vi "串口数据采集.vi"() -> ()   [LabVIEW 2014]
uses:
  <vilib>/Instr/_visa.llb/VISA Configure Serial Port (Instr).vi
panel:
  out "帮助文档":string="               系统使用说明\n     欢迎使用LabVIEW温度监控系统V3.0！\n      ①程序运行时此帮助文档5秒后会自动关闭。\n      ②程序运行前请先正确配置串口号。\n      ③采样周期默认为1000ms，可根据需要在线设置，但建议不低于500。\n      ④状态及数据区显示系统运行的各种状态或采集的原始数据；时间记录区显示的分别是系统已运行的时间及系统开始运行的起始时刻。\n      ⑤默认的温度上下限分别为25℃和15℃，可随时根据实际情况修改，温度超过设定界限对应指示灯会闪烁并伴有蜂鸣器警告。\n      ⑥设置的快捷键：串口开关按钮<Shift+F1>,帮助按钮<Home>，停止按钮<End>，退出按钮<Delete>。\n      \n"
  in  "帮助":bool
  in  "退出":bool
  in  "停止":bool
  out "状态及数据":string="程序待运行……"
  out "数据采集量":dbl format="%06.0f"
  out "0CH":dbl format="%.2g"
  out "1CH":dbl format="%.2f"
  out "2CH":dbl format="%.2g"
  out "运行时间":string="0  00:00:00"
  out "开始时刻":string="2017/1/1 00:00:00"
  out "低温":bool
  out "高温":bool
  out "2CH":bool
  out "1CH":bool
  out "0CH":bool
  in  "串口开关":bool
  in  "低温限":dbl=15.0 format="%.1g"
  in  "高温限":dbl=25.0 format="%.1f"
  in  "起始号":dbl format="%0#6.0p"
  in  "周期":u32=1000
  in  "端口":refnum<visa-resource-name>="COM2" caption="端口号"
  out "温度曲线":dynamicdata(graph)
  # "LabVIEW温度监控系统V3.0"
  # "串口配置"
  # "采样周期"
  # "时间记录"
  # "数据采集量"
  # "超限报警"
  # "状态及数据"
  # "数值显示"
  # "退出"
  # "停止"
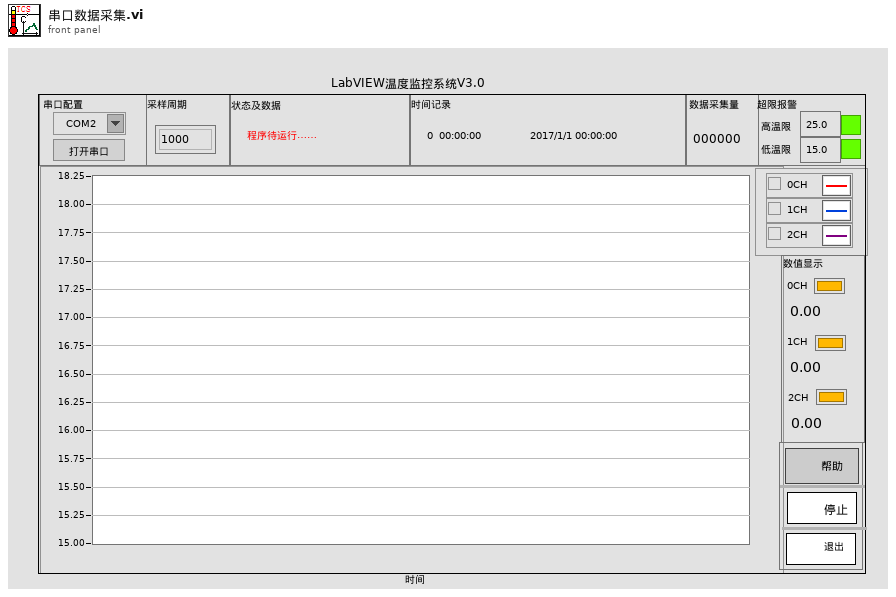
[diagram p1: front panel]
types:
  T1 = enum8{"Enabled", "Disabled", "Disabled and Grayed Out"}
  T2 = enum16{"open", "replace", "create", "open or create", "replace or create", "replace or create with confirmation"}
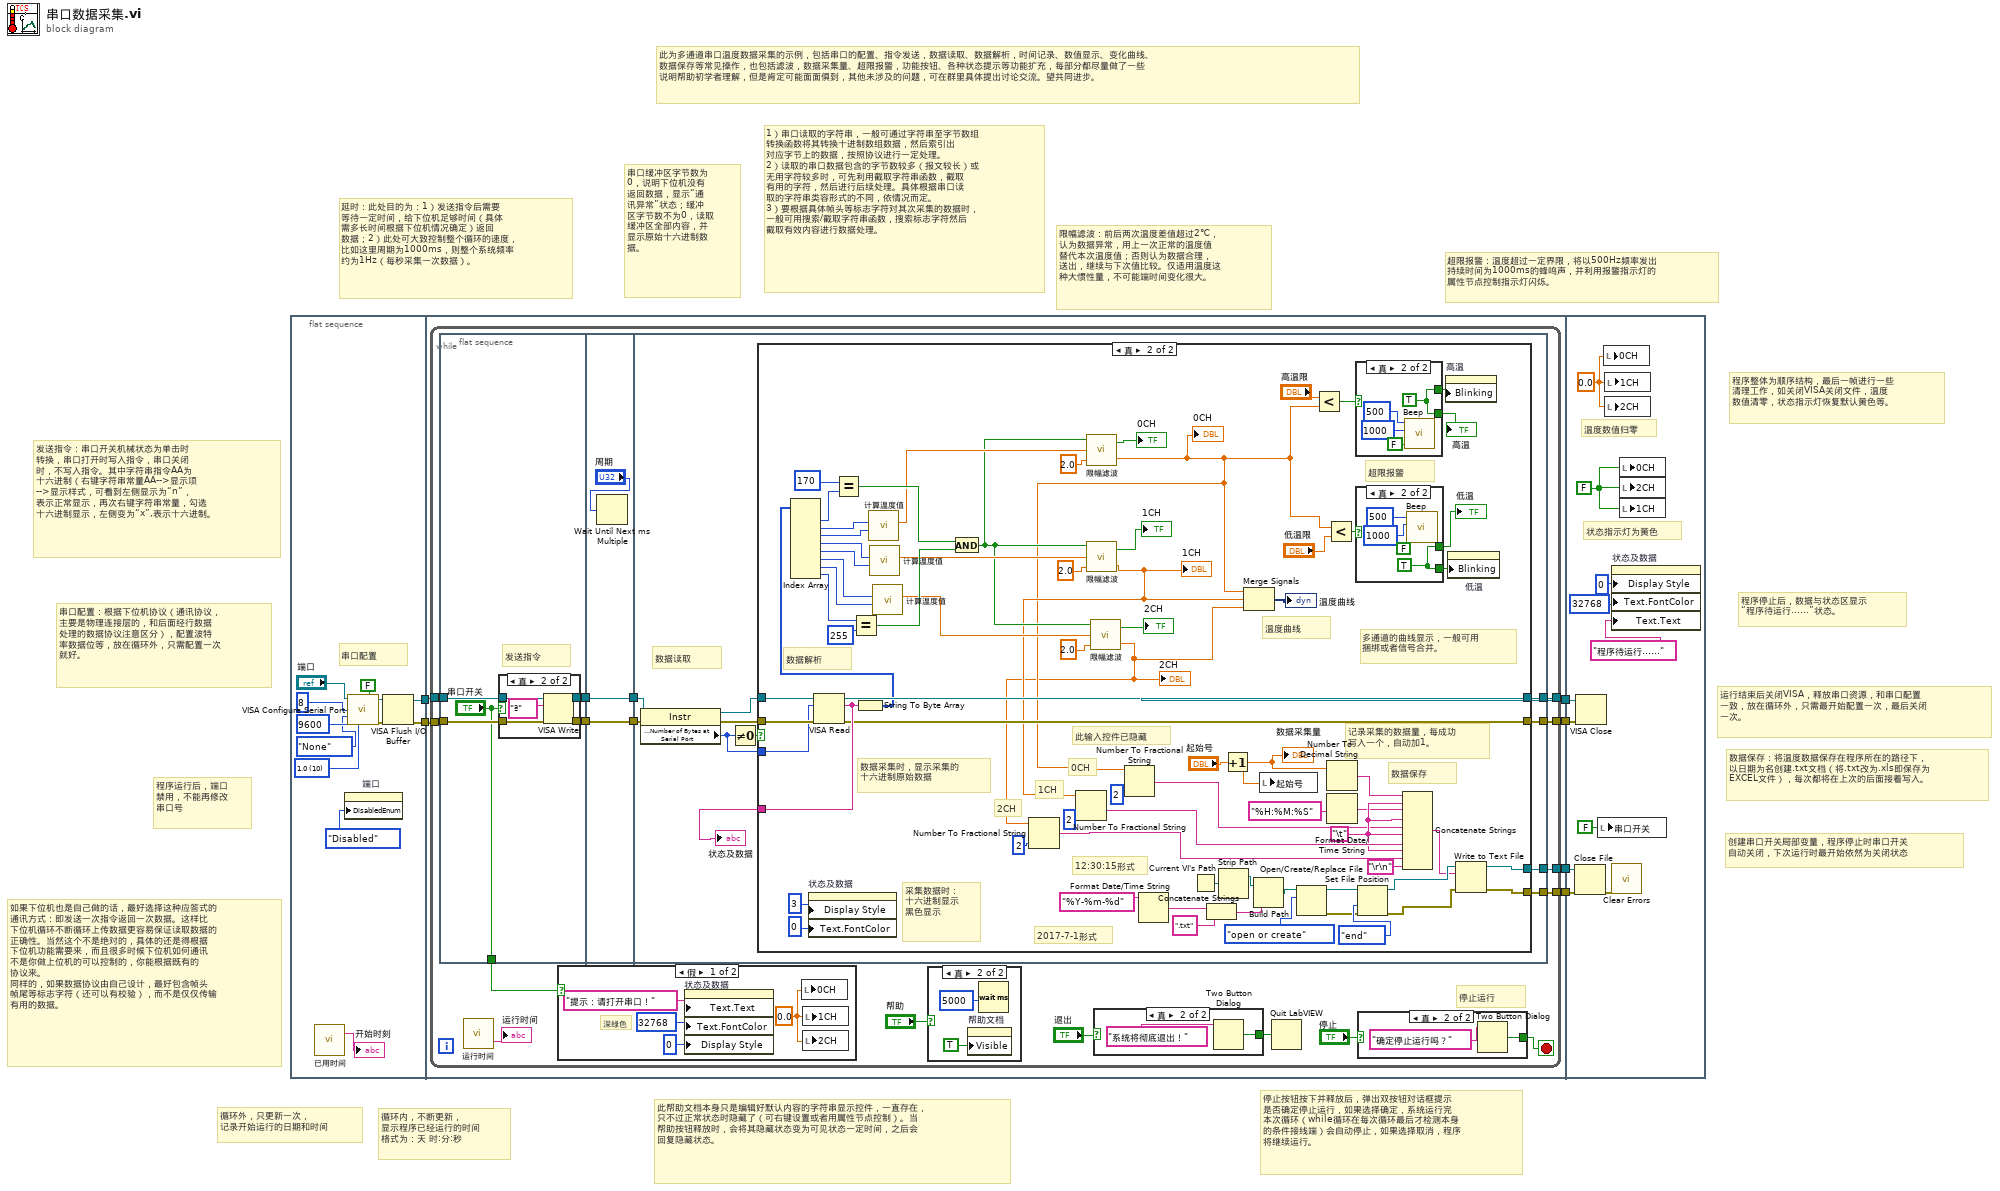
[diagram p0: block diagram]
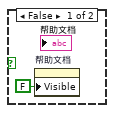
[diagram p2: hidden frame]
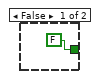
[diagram p3: hidden frame]
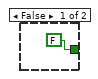
[diagram p5: hidden frame]
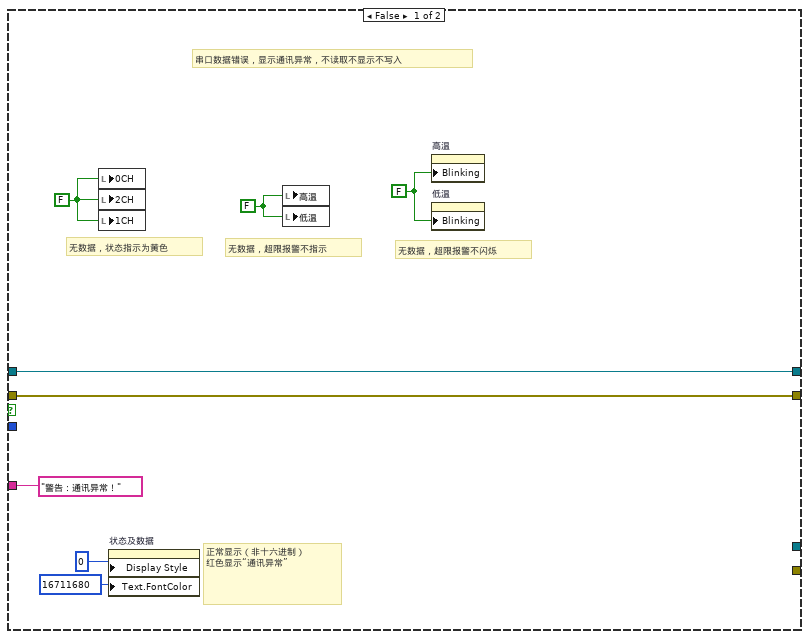
[diagram p7: hidden frame]
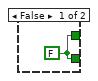
[diagram p8: hidden frame]
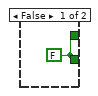
[diagram p9: hidden frame]
diagram:
  # "此为多通道串口温度数据采集的示例，包括串口的配置、指令发送，数据读取、数据解析，时间记录、数值显示、变化曲线、\n数据保存等常见操作，也包括滤波，数据采集量、超限报警，功能按钮、各种状态提示等功能扩充，每部分都尽量做了一些\n说明帮助初学者理解，但是肯定可能面面俱到，其他未涉及的问题，可在群里具体提出讨论交流。望共同进步。"
  # "程序整体为顺序结构，最后一帧进行一些\n清理工作，如关闭VISA关闭文件，温度\n数值清零，状态指示灯恢复默认黄色等。"
  # "创建串口开关局部变量，程序停止时串口开关\n自动关闭，下次运行时最开始依然为关闭状态"
  # "如果下位机也是自己做的话，最好选择这种应答式的\n通讯方式：即发送一次指令返回一次数据。这样比\n下位机循环不断循环上传数据更容易保证读取数据的\n正确性。当然这个不是绝对的，具体的还是得根据\n下位机功能需要来，而且很多时候下位机如何通讯\n不是你做上位机的可以控制的，你能根据既有的\n协议来。\n同样的，如果数据协议由自己设计，最好包含帧头\n帧尾等标志字符（还可以有校验），而不是仅仅传输\n有用的数据。"
  # "1）串口读取的字符串，一般可通过字符串至字节数组\n转换函数将其转换十进制数组数据，然后索引出\n对应字节上的数据，按照协议进行一定处理。\n2）读取的串口数据包含的字节数较多（报文较长）或\n无用字符较多时，可先利用截取字符串函数，截取\n有用的字符，然后进行后续处理。具体根据串口读\n取的字符串类容形式的不同，依情况而定。\n3）要根据具体帧头等标志字符对其次采集的数据时，\n一般可用搜索/截取字符串函数，搜索标志字符然后\n截取有效内容进行数据处理。"
  # "程序停止后，数据与状态区显示\n“程序待运行……”状态。"
  # "串口缓冲区字节数为\n0，说明下位机没有\n返回数据，显示“通\n讯异常”状态；缓冲\n区字节数不为0，读取\n缓冲区全部内容，并\n显示原始十六进制数\n据。"
  # "运行结束后关闭VISA，释放串口资源，和串口配置\n一致，放在循环外，只需最开始配置一次，最后关闭\n一次。"
  # "数据保存：将温度数据保存在程序所在的路径下，\n以日期为名创建.txt文档（将.txt改为.xls即保存为\nEXCEL文件），每次都将在上次的后面接着写入。"
  # "超限报警：温度超过一定界限，将以500Hz频率发出\n持续时间为1000ms的蜂鸣声，并利用报警指示灯的\n属性节点控制指示灯闪烁。"
  # "停止按钮按下并释放后，弹出双按钮对话框提示\n是否确定停止运行，如果选择确定，系统运行完\n本次循环（while循环在每次循环最后才检测本身\n的条件接线端）会自动停止，如果选择取消，程序\n将继续运行。"
  # "此帮助文档本身只是编辑好默认内容的字符串显示控件，一直存在，\n只不过正常状态时隐藏了（可右键设置或者用属性节点控制）。当\n帮助按钮释放时，会将其隐藏状态变为可见状态一定时间，之后会\n回复隐藏状态。"
  # "延时：此处目的为：1）发送指令后需要\n等待一定时间，给下位机足够时间（具体\n需多长时间根据下位机情况确定）返回\n数据；2）此处可大致控制整个循环的速度，\n比如这里周期为1000ms，则整个系统频率\n约为1Hz（每秒采集一次数据）。"
  # "发送指令：串口开关机械状态为单击时\n转换，串口打开时写入指令，串口关闭\n时，不写入指令。其中字符串指令AA为\n十六进制（右键字符串常量AA-->显示项\n-->显示样式，可看到左侧显示为“n”，\n表示正常显示，再次右键字符串常量，勾选\n十六进制显示，左侧变为“x”,表示十六进制。"
  # "串口配置：根据下位机协议（通讯协议，\n主要是物理连接层的，和后面经行数据\n处理的数据协议注意区分），配置波特\n率数据位等，放在循环外，只需配置一次\n就好。"
  # "程序运行后，端口\n禁用，不能再修改\n串口号"
  # "限幅滤波：前后两次温度差值超过2℃，\n认为数据异常，用上一次正常的温度值\n替代本次温度值；否则认为数据合理，\n送出，继续与下次值比较。仅适用温度这\n种大惯性量，不可能端时间变化很大。"
  # "循环内，不断更新，\n显示程序已经运行的时间\n格式为：天 时:分:秒"
  # "循环外，只更新一次，\n记录开始运行的日期和时间"
  n1 = flat-sequence {
    tunnel: [w12] -> w6
    tunnel: [w13] -> w5
    tunnel: w6 -> [w24]
    tunnel: w5 -> [w23]
    tunnel: [w22] -> w4
    tunnel: [w21] -> w3
    tunnel: [w20] -> w2
    tunnel: [w19] -> w1
    tunnel: w4 -> [w180]
    tunnel: w3 -> [w181]
    tunnel: w2 -> [w179]
    tunnel: w1 -> [w178]
    frame #0 {
      w9 = u16 10 items=["1.0"=10, "1.5"=15, "2.0"=20] ("stop bits (10: 1 bit)")
      # "串口配置"
      n2 = call "已用时间"() -> ("Present Text"=→"开始时刻":string)  [unwired: 12 in, 7 out]
      n3 = property on="端口" class="VISAName"("DisabledEnum"=T1."Disabled" ("禁用")) -> ()  [unwired: 2 in, 2 out]
      n4 = call-poly "VISA Configure Serial Port"("VISA resource name"="端口", "Enable Termination\nChar (T)"=FALSE ("Enable Termination\nChar (T)"), "baud rate (9600)"=u32 9600, "data bits (8)"=u16 8, "parity (0:none)"=enum16{"None", "Odd", "Even", "Mark", "Space"}."None", "stop bits (10: 1 bit)"=w9) -> ("VISA resource name out"=w14:refnum<visa-resource-name>, "error out"=w15:errorcluster)  [unwired: 8 in]
      n5 = VISA Flush I/O Buffer(VISA resource name=w14, error in (no error)=w15) -> (VISA resource name out=w12:refnum<visa-resource-name>, error out=w13:errorcluster)  [unwired: 1 in]
    }
    frame #1 {
      n6 = while {
        tunnel: w24 -> [w37]
        tunnel: w23 -> [w36]
        tunnel: [w35] -> w22
        tunnel: [w34] -> w21
        tunnel: [w32] -> w20
        tunnel: [w31] -> w19
        stop <- w33 stop-if-true
        # "停止运行"
        # "下位机数据帧格式0xAA 0xXX 0xXX  0xXX 0xXX 0xXX 0xXX 0xFF"
        n7 = flat-sequence {
          tunnel: [w59] -> w41
          tunnel: [w58] -> w40
          tunnel: w37 -> [w57]
          tunnel: w36 -> [w56]
          tunnel: ["串口开关"] -> w30
          tunnel: w41 -> [w69]
          tunnel: w40 -> [w68]
          tunnel: [w69] -> w39
          tunnel: [w68] -> w38
          tunnel: w39 -> [w79]
          tunnel: w38 -> [w78]
          tunnel: [w80] -> w34
          tunnel: [w75] -> w35
          tunnel: [w73] -> w32
          tunnel: [w72] -> w31
          frame #0 {
            # "发送指令"
            n8 = case shown="真" "串口开关" {
              tunnel: [w61 w66] -> w59
              tunnel: [w60 w65] -> w58
              tunnel: w57 -> [w61 w64]
              tunnel: w56 -> [w60 w63]
              frame False {
              }
              frame True {
                n9 = VISA Write(VISA resource name=w64, write buffer="ª" ("写入缓冲区"), error in (no error)=w63) -> (VISA resource name out=w66:refnum<visa-resource-name>, error out=w65:errorcluster)  [unwired: 1 out]
              }
            }
          }
          frame #1 {
            n10 = Wait Until Next ms Multiple(millisecond multiple="周期") -> ()  [unwired: 1 out]
          }
          frame #2 {
            # "数据读取"
            n11 = property class="Instr"(reference=w79, error in=w78) -> (reference out=w77:refnum<visa-resource-name>, error out=w76:errorcluster, "Serial Settings:Number of Bytes at Serial Port"=w74:u32)
            n12 = Not Equal To 0?(x=w74) -> (x != 0?=w71:bool)
            n13 = case shown="真" w71 {
              tunnel: [w87 w115] -> w80
              tunnel: w77 -> [w88 w160]
              tunnel: w76 -> [w87 w159]
              tunnel: [w88 w158] -> w75
              tunnel: w74 -> [_ w156]
              tunnel: [_ w130] -> w73
              tunnel: [_ w129] -> w72
              tunnel: ["警告：通讯异常！" w125] -> w70
              frame False {
                w83 = FALSE ("2CH")
                w84 = FALSE ("2CH")
                w85 = FALSE ("2CH")
                # "正常显示（非十六进制）\n红色显示“通讯异常”"
                # "无数据，超限报警不闪烁"
                # "无数据，超限报警不指示"
                # "无数据，状态指示为黄色"
                # "串口数据错误，显示通讯异常，不读取不显示不写入"
                n14 = local write "0CH"(w85) -> ()
                n15 = local write "2CH"(w85) -> ()
                n16 = local write "1CH"(w85) -> ()
                n17 = property on="状态及数据" class="Str"("Display Style"=u32 0 ("显示样式"), "Text.FontColor"=u32 16711680 ("文本.字体:颜色")) -> ()  [unwired: 2 in, 2 out]
                n18 = local write "高温"(w84) -> ()
                n19 = local write "低温"(w84) -> ()
                n20 = property on="高温" class="Bool (严格)"("Blinking"=w83) -> ()  [unwired: 2 in, 2 out]
                n21 = property on="低温" class="Bool (严格)"("Blinking"=w83) -> ()  [unwired: 2 in, 2 out]
              }
              frame True {
                w120 = "\t"
                # "此输入控件已隐藏"
                # "记录采集的数据量，每成功\n写入一个，自动加1。"
                # "12:30:15形式"
                # "2017-7-1形式"
                # "多通道的曲线显示，一般可用\n捆绑或者信号合并。"
                # "数据采集时，显示采集的\n十六进制原始数据"
                # "2CH"
                # "1CH"
                # "0CH"
                # "数据解析"
                # "采集数据时：\n十六进制显示\n黑色显示"
                # "温度曲线"
                # "超限报警"
                # "数据保存"
                n22 = property on="状态及数据" class="Str"("Display Style"=u32 3 ("显示样式"), "Text.FontColor"=u32 0 ("文本.字体:颜色")) -> ()  [unwired: 2 in, 2 out]
                n23 = VISA Read(VISA resource name=w160, byte count=w156, error in (no error)=w159) -> (VISA resource name out=w158:refnum<visa-resource-name>, read buffer=w125:string, error out=w115:errorcluster)  [unwired: 1 out]
                n24 = String To Byte Array(string=w125) -> (unsigned byte array=w157:u8[])
                n25 = Index Array(array=w157) -> (element #1=w149:u8, element #2=w154:u8, element #3=w153:u8, element #4=w152:u8, element #5=w151:u8, element #6=w124:u8, element #7=w123:u8, element #8=w122:u8)  [unwired: 8 in]
                n26 = Equal?(x=u8 170 ("元素"), y=w149) -> (x = y?=w147:bool)
                n27 = Equal?(x=w122, y=u8 255) -> (x = y?=w116:bool)
                n28 = call "计算温度值.vi"("数值L"=w153, "数值H"=w154) -> ("温度数值"=w103:dbl)  [unwired: 9 in]
                n29 = call "计算温度值.vi"("数值L"=w151, "数值H"=w152) -> ("温度数值"=w100:dbl)  [unwired: 9 in]
                n30 = call "计算温度值.vi"("数值L"=w123, "数值H"=w124) -> ("温度数值"=w97:dbl)  [unwired: 9 in]
                n31 = And(x=w147, y=w116) -> (x .and. y?=w96:bool)
                n32 = call "限幅滤波.vi"("限幅值"=2.0 ("y"), "输入值"=w103, "校验结果"=w96) -> ("输出值"=w92:dbl, "状态指示"=→"0CH":bool)  [unwired: 1 in]
                "0CH" <- w92
                n33 = call "限幅滤波.vi"("限幅值"=2.0 ("y"), "输入值"=w100, "校验结果"=w96) -> ("输出值"=w93:dbl, "状态指示"=→"1CH":bool)  [unwired: 1 in]
                "1CH" <- w93
                n34 = Number To Fractional String(number=w93, precision (6)=i16 2 ("精度(6)")) -> (F-format string=w133:string)  [unwired: 2 in]
                n35 = call "限幅滤波.vi"("限幅值"=2.0 ("y"), "输入值"=w97, "校验结果"=w96) -> ("输出值"=w91:dbl, "状态指示"=→"2CH":bool)  [unwired: 1 in]
                "2CH" <- w91
                n36 = Number To Fractional String(number=w91, precision (6)=i16 2 ("精度(6)")) -> (F-format string=w132:string)  [unwired: 2 in]
                n37 = Number To Fractional String(number=w92, precision (6)=i16 2 ("精度(6)")) -> (F-format string=w117:string)  [unwired: 2 in]
                n38 = Format Date/Time String(time format string (%c)="%Y-%m-%d" ("时间格式字符串(%c)")) -> (date/time string=w139:string)  [unwired: 2 in]
                n39 = Current VI's Path() -> (path=w137:path)
                n40 = Concatenate Strings(w139, ".txt" ("名称或相对路径")) -> (w142:string)
                n41 = Strip Path(path=w137) -> (stripped path=w138:path)  [unwired: 1 out]
                n42 = Increment(x="起始号") -> (x+1=w106:dbl)
                "数据采集量" <- w106
                n43 = Merge Signals ("合并信号")(w92, w93, w91) -> (→"温度曲线":dynamicdata)
                n44 = Build Path(base path=w138, name or relative path=w142) -> (appended path=w144:path)
                n45 = local write "起始号"(w106) -> ()
                n46 = Open/Create/Replace File(file path (use dialog)=w144, operation (0:open)=T2."open or create" ("操作(0:open)")) -> (refnum out=w141:refnum<file>, error out=w89:errorcluster)  [unwired: 4 in, 1 out]
                n47 = Less?(x="高温限", y=w92) -> (x < y?=w112:bool)
                n48 = Less?(x=w92, y="低温限") -> (x < y?=w111:bool)
                n49 = Number To Decimal String(number=w106) -> (decimal integer string=w121:string)  [unwired: 1 in]
                n50 = Format Date/Time String(time format string (%c)="%H:%M:%S" ("时间格式字符串(%c)")) -> (date/time string=w119:string)  [unwired: 2 in]
                n51 = case shown="真" w112 {
                  tunnel: [w166 w167] -> w110
                  tunnel: [w166 w167] -> w108
                  frame False {
                    w166 = FALSE
                  }
                  frame True {
                    w167 = TRUE
                    n52 = call <vilib>:"Beep.vi"("use system alert? (T)"=FALSE, "duration (msec)"=u32 1000, "frequency (Hz)"=u32 500) -> ()  [unwired: 9 in]
                  }
                }
                "高温" <- w110
                n53 = case shown="真" w111 {
                  tunnel: [w161 w162] -> w109
                  tunnel: [w161 w162] -> w107
                  frame False {
                    w161 = FALSE
                  }
                  frame True {
                    w162 = TRUE
                    n54 = call <vilib>:"Beep.vi"("use system alert? (T)"=FALSE, "duration (msec)"=u32 1000, "frequency (Hz)"=u32 500) -> ()  [unwired: 9 in]
                  }
                }
                "低温" <- w109
                n55 = Set File Position(refnum=w141, from (0:start)=enum16{"start", "end", "current"}."end" ("自（0:起始）"), error in=w89) -> (refnum out=w136:refnum<file>, error out=w90:errorcluster)  [unwired: 1 in]
                n56 = Concatenate Strings(w121, w120, w119, w120, w117, w120, w133, w120, w132, "\r\n") -> (w128:string)
                n57 = property on="高温" class="Bool (严格)"("Blinking"=w108) -> ()  [unwired: 2 in, 2 out]
                n58 = property on="低温" class="Bool (严格)"("Blinking"=w107) -> ()  [unwired: 2 in, 2 out]
                n59 = Write to Text File(file (use dialog)=w136, text=w128, error in=w90) -> (refnum out=w130:refnum<file>, error out=w129:errorcluster)  [unwired: 1 in, 1 out]
              }
            }
            "状态及数据" <- w70
          }
        }
        n60 = call "运行时间"() -> ("Elapsed Time Text"=→"运行时间":string)  [unwired: 12 in, 7 out]
        n61 = case shown="假" w30 {
          frame False {
            w49 = 0.0 ("1CH")
            # "深绿色"
            n62 = property on="状态及数据" class="Str"("Text.Text"="提示：请打开串口！" ("文本.文本"), "Text.FontColor"=u32 32768 ("文本.字体:颜色"), "Display Style"=u32 0 ("显示样式")) -> ()  [unwired: 2 in, 2 out]
            n63 = local write "0CH"(w49) -> ()
            n64 = local write "1CH"(w49) -> ()
            n65 = local write "2CH"(w49) -> ()
          }
          frame True {
          }
        }
        n66 = case shown="真" "帮助" {
          frame False {
            n67 = property on="帮助文档" class="Str"("Visible"=FALSE ("可见")) -> ()  [unwired: 2 in, 2 out]
          }
          frame True {
            n68 = property on="帮助文档" class="Str"("Visible"=TRUE ("可见")) -> ()  [unwired: 2 in, 2 out]
            n69 = Wait (ms)(milliseconds to wait=u32 5000 ("等待时间（毫秒）")) -> ()  [unwired: 1 out]
          }
        }
        n70 = case shown="真" "退出" {
          tunnel: [FALSE ("T button?") w46] -> w29
          frame False {
          }
          frame True {
            n71 = Two Button Dialog(message="系统将彻底退出！" ("消息")) -> (T button?=w46:bool)  [unwired: 2 in]
          }
        }
        n72 = Quit LabVIEW(quit? (T)=w29) -> ()
        n73 = case shown="真" "停止" {
          tunnel: [FALSE ("T button?") w53] -> w33
          frame False {
          }
          frame True {
            n74 = Two Button Dialog(message="确定停止运行吗？" ("消息")) -> (T button?=w53:bool)  [unwired: 2 in]
          }
        }
      }
    }
    frame #2 {
      w171 = FALSE ("2CH")
      w176 = 0.0 ("1CH")
      # "状态指示灯为黄色"
      # "温度数值归零"
      n75 = Close File(refnum=w179, error in=w178) -> (error out=w172:errorcluster)  [unwired: 1 out]
      n76 = VISA Close(VISA resource name=w180, error in (no error)=w181) -> ()  [unwired: 1 out]
      n77 = local write "串口开关"(FALSE) -> ()
      n78 = local write "0CH"(w176) -> ()
      n79 = local write "1CH"(w176) -> ()
      n80 = local write "2CH"(w176) -> ()
      n81 = property on="状态及数据" class="Str"("Display Style"=u32 0 ("显示样式"), "Text.FontColor"=u32 32768 ("文本.字体:颜色"), "Text.Text"="程序待运行……" ("文本.文本")) -> ()  [unwired: 2 in, 2 out]
      n82 = call <vilib>:"Clear Errors.vi"("error in (no error)"=w172) -> ()  [unwired: 5 in, 2 out]
      n83 = local write "0CH"(w171) -> ()
      n84 = local write "2CH"(w171) -> ()
      n85 = local write "1CH"(w171) -> ()
    }
  }
